vi "Start.vi"(8 "error in (no error)":errorcluster, 10 "Params":variant, 11 "FitterBase in":refnum<class "FitterBase.lvclass">) -> (0 "error out":errorcluster, 3 "FitterBase out":refnum<class "FitterBase.lvclass">)   [LabVIEW 2018, in "AnalysisPlugins.lvlib" / "FitterBase.lvclass"]
uses:
  FitterBase.lvclass
  AnalysisPluginBaseClass/AnalysisPluginsBase.lvclass
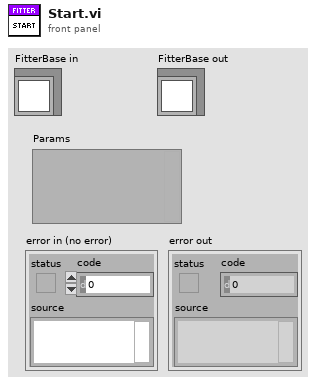
[diagram p1: front panel]
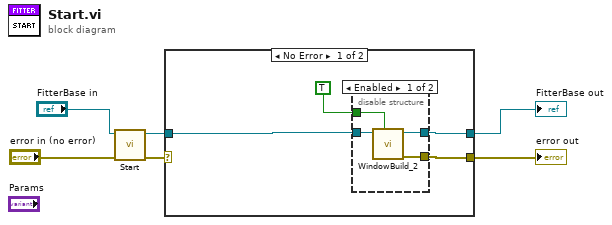
[diagram p0: block diagram]
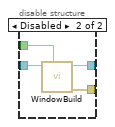
[diagram p2: hidden frame]
diagram:
  n1 = call-parent "Start.vi"("error in (no error)"="error in (no error)", "AnalysisPluginsBase in"="FitterBase in") -> ("error out"=w4:errorcluster, "AnalysisPluginsBase out"=w3:refnum<class "FitterBase.lvclass">)  [unwired: 8 in]
  n2 = case shown="No Error" w4 {
    selector: w4 -> [_ w19]
    tunnel: w3 -> [w10 w20]
    tunnel: [w8 w20] -> w2
    tunnel: [w7 w19] -> w1
    frame No Error {
      n3 = disable-structure shown="Enabled" {
        disable-tunnel: w10 -> [w14 w18]
        disable-tunnel: TRUE ("Start") -> [w13 w15]
        disable-tunnel: [w12 w17] -> w8
        disable-tunnel: [w11 w16] -> w7
        frame Enabled {
          n4 = call "WindowBuild_2.vi"("Init"=w13, "Fitter in"=w14) -> ("Error Out"=w11:errorcluster, "Fitter out"=w12:refnum<class "FitterBase.lvclass">)  [unwired: 7 in, 1 out]
        }
        frame Disabled {
          n5 = call "WindowBuild.vi"("Init"=w15, "Fitter in"=w18) -> ("error out"=w16:errorcluster, "Fitter out"=w17:refnum<class "FitterBase.lvclass">)  [unwired: 7 in, 1 out]
        }
      }
    }
    frame Error {
    }
  }
  "error out" <- w1
  "FitterBase out" <- w2
